vi "Timestamp to Unix Epoch.vi"(11 "seconds since 1Jan1904":timestamp) -> (3 "String":string)   [LabVIEW 2026, in "TALOS.lvlib"]
uses:
  TALOS.lvlib
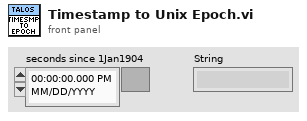
[diagram p1: front panel]
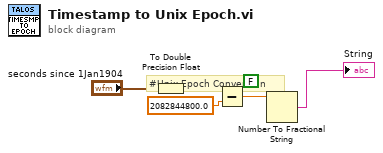
[diagram p0: block diagram]
diagram:
  # "#Unix-Epoch Conversion"
  n1 = To Double Precision Float(number="seconds since 1Jan1904") -> (double precision float=w3:dbl)
  n2 = Subtract(x=w3, y=2082844800.0) -> (x-y=w4:dbl)
  n3 = Number To Fractional String(use system decimal point (T)=FALSE, number=w4) -> (F-format string=→"String":string)  [unwired: 2 in]
